vi "define.vi"(8 "error in (no error)":errorcluster, 11 "TrajectoryAK101022Resonance in":refnum<class "TrajectoryAK101022Resonance.lvclass">) -> (0 "error out":errorcluster, 3 "TrajectoryAK101022Resonance out":refnum<class "TrajectoryAK101022Resonance.lvclass">)   [LabVIEW 2010, in "TrajectoryAK101022Resonance.lvclass"]
doc: "modal dialog on which the user can set the trajectory parameters"
uses:
  TrajectoryAK101022Resonance.lvclass
  filter_type_enum.ctl
  TrajectoryAK101022Resonance.lvclass/TrajectoryAK101022Resonance.ctl
panel:
  out "frame rate":dbl[unit]
  out "resonance frequency":dbl[unit]
  out "Number of z points":i32
  out "repetitions (volumes)":i32
  out "number of planes":i32
  out "step size":dbl[unit]
  out "z signal":dbl[unit][][](graph)
  in  "Filter on?":bool
  in  "z-Function type":enum32{"Sine", "Stack", "Step"}(tab)
  out "ETL frequency":dbl[unit]=1.0 min=1.0
  in  "ETL amplitude conversion":dbl[unit]=500.0
  in  "ETL phase delay":dbl[unit]=0.008726646259971648
  in  "bi-directional?":bool
  in  "angle fraction":dbl=0.5
  out "Lines per z step (sine)":i32=1 caption="lines per z step" min=1
  in  "Level High (Step)":dbl caption="Level High"
  in  "Lines per z step (Step)":i32 caption="Lines per z step" min=1
  in  "Level overshoot (Step)":dbl caption="Level overshoot"
  in  "Level undershoot (Step)":dbl caption="Level undershoot"
  in  "Sample level high (Step)":u16 caption="Sample level high"
  in  "Sample overshoot (Step)":u16 caption="Sample overshoot"
  in  "Sample ramp (Step)":u16 caption="Sample ramp"
  in  "Sample undershoot (Step)":u16 caption="Sample undershoot"
  in  "filter type":T1
  in  "filter order":u16=2
  in  "low cutoff freq":dbl=0.125
  in  "high cutoff freq":dbl=0.45
  in  "button:cancel":bool
  in  "button:ok":bool
  # "Define TrajectoryAK101022Resonance"
  # "Filtering"
  # "In this mode, the z signal is sine function."
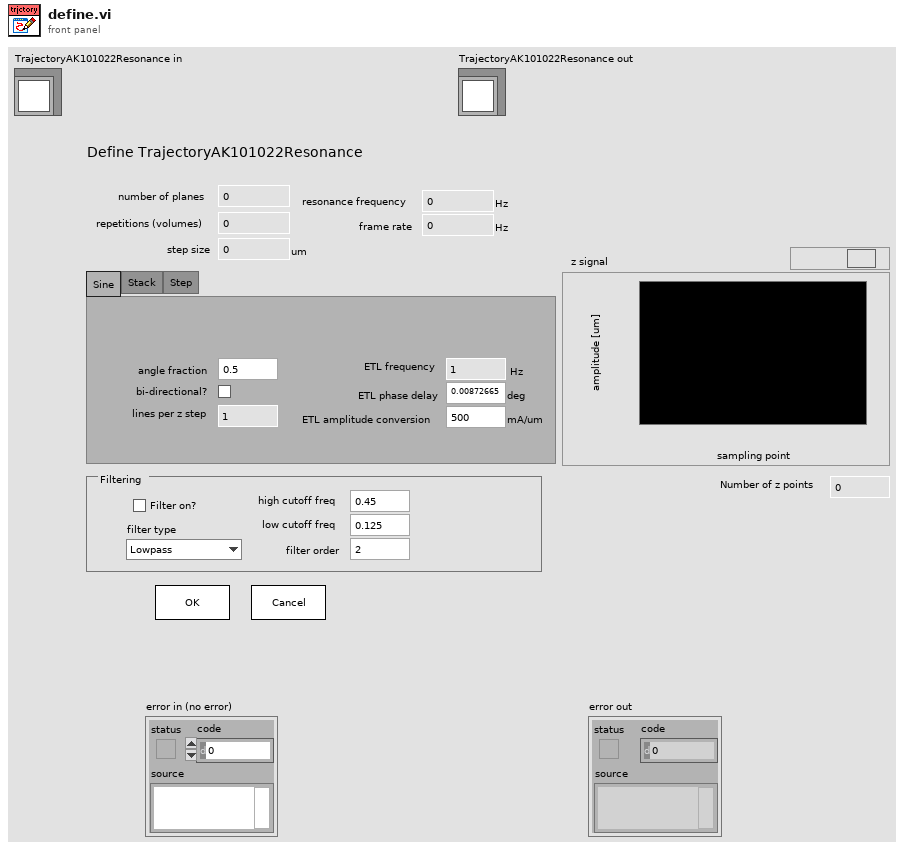
[diagram p1: front panel]
types:
  T1 = typedef "TrajectoryAK101022Resonance.lvclass/filter_type_enum.ctl" = enum16{"Lowpass", "Highpass", "Bandpass", "Bandstop"}
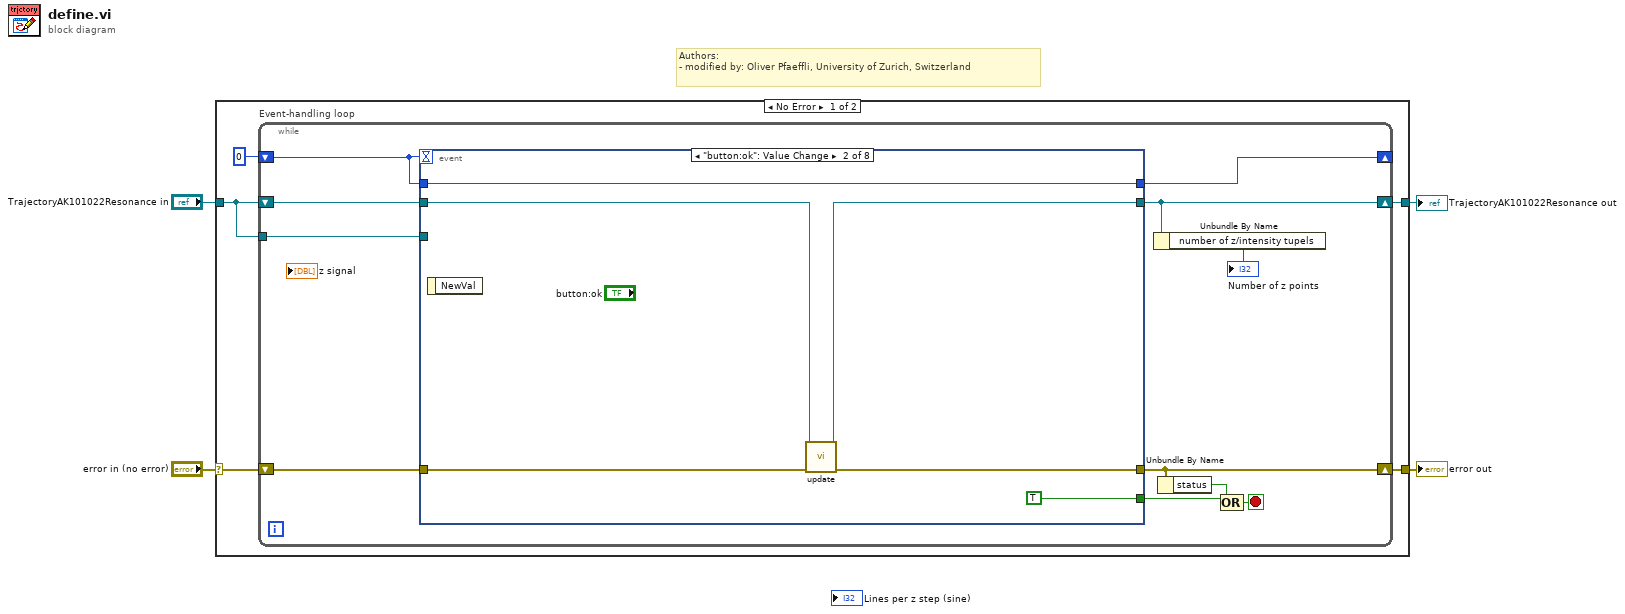
[diagram p0: block diagram]
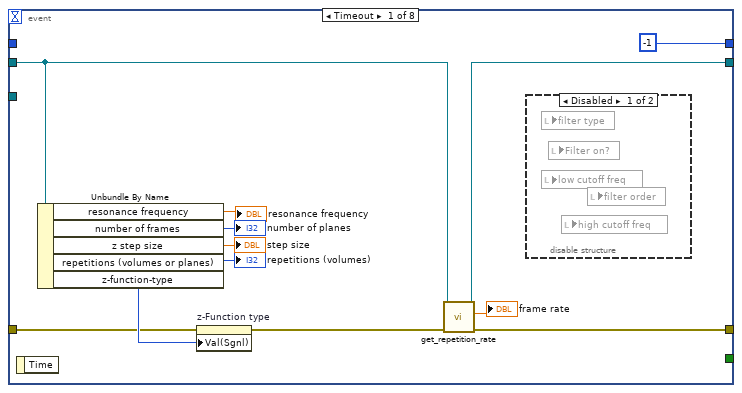
[diagram p2: hidden frame]
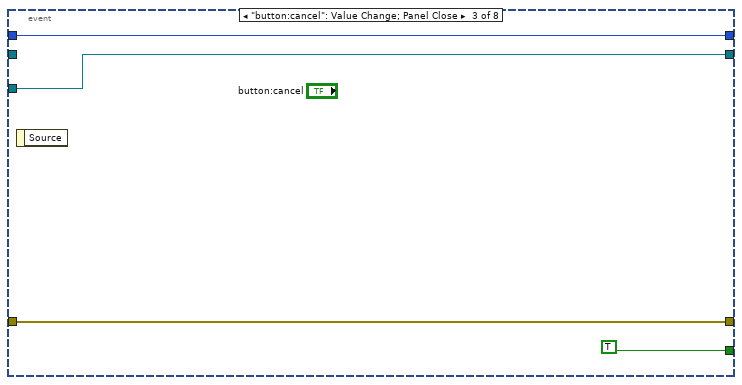
[diagram p4: hidden frame]
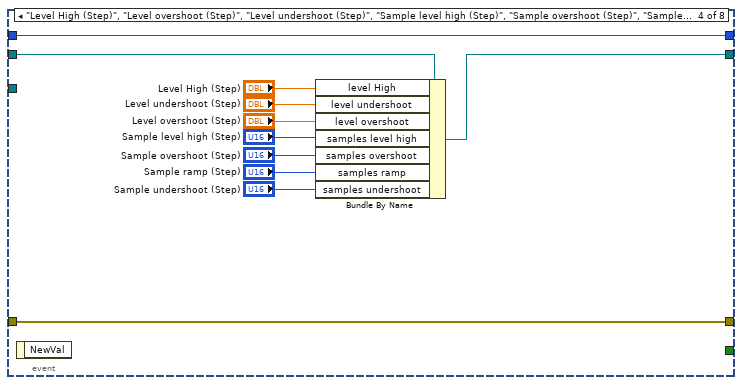
[diagram p5: hidden frame]
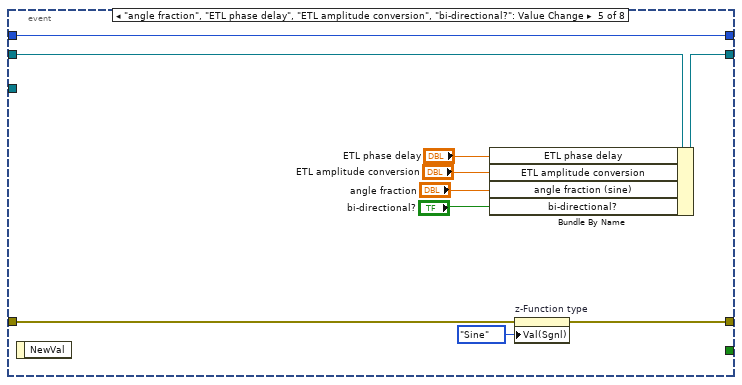
[diagram p6: hidden frame]
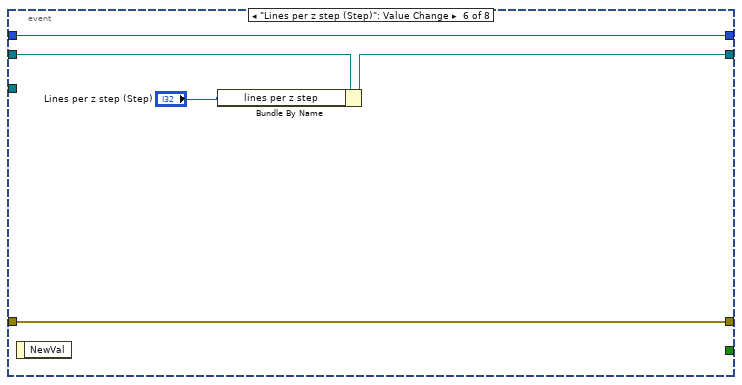
[diagram p7: hidden frame]
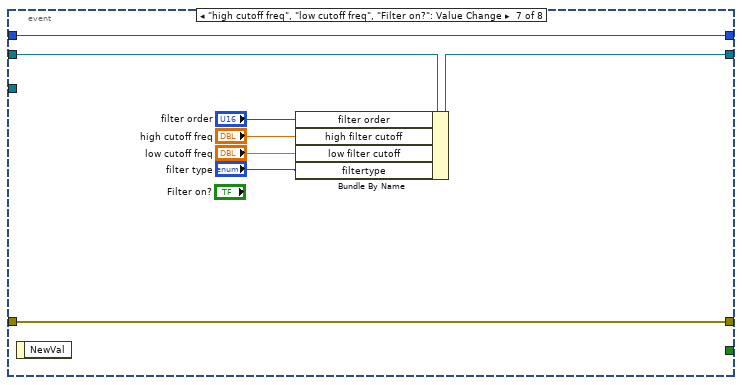
[diagram p8: hidden frame]
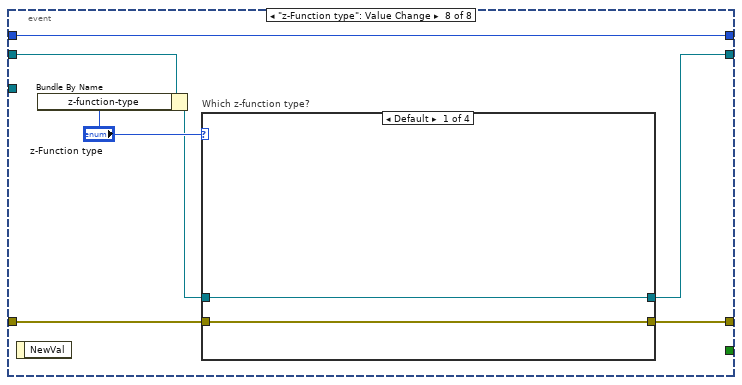
[diagram p9: hidden frame]
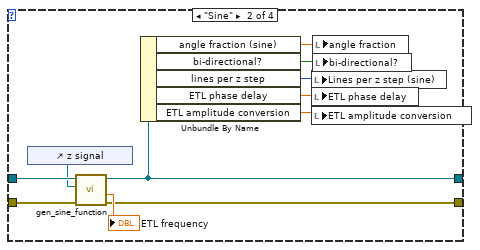
[diagram p10: hidden frame]
diagram:
  # "Authors: \n- modified by: Oliver Pfaeffli, University of Zurich, Switzerland"
  n1 = case shown="No Error" "error in (no error)" {
    selector: "error in (no error)" -> [w9 w102]
    tunnel: [w8 w102] -> w3
    tunnel: "TrajectoryAK101022Resonance in" -> [w5 w101]
    tunnel: [w7 w101] -> w1
    frame No Error {
      n2 = while "Event-handling loop" {
        shift-right: [w13] -> w8
        shift-left: w9 -> [w14]
        shift-right: [w16] -> _
        shift-left: 0 -> [w17]
        shift-right: [w11] -> w7
        shift-left: w5 -> [w18]
        tunnel: w5 -> [w15]
        stop <- w19 stop-if-true
        n3 = event shown="[1] \"button:ok\": Value Change" {
          selector: _ -> [_ _ _ _ _ _ _ _]
          dyn-events: _ -> [_ _ _ _ _ _ _ _]
          timeout: w17 -> [_ _ _ _ _ _ _ _]
          tunnel: w18 -> [w24 w33 _ w52 w54 w67 w75 w83]
          tunnel: w17 -> [_ w38 w42 w43 w63 w64 w69 w77]
          tunnel: [-1 w38 w42 w43 w63 w64 w69 w77] -> w16
          tunnel: [w27 w36 w41 w51 w62 w66 w74 w78] -> w11
          tunnel: w15 -> [_ _ w41 _ _ _ _ _]
          tunnel: w14 -> [w22 w34 w40 w53 w55 w68 w76 w82]
          tunnel: [w26 w35 w40 w53 w57 w68 w76 w81] -> w13
          tunnel: [_ TRUE TRUE _ _ _ _ _] -> w12
          event Timeout {
            n4 = event-data() -> ()  [unwired: 1 in, 1 out]
            n5 = Unbundle By Name(w24) -> ("resonance frequency"=→"resonance frequency":dbl[unit], "number of frames"=→"number of planes":i32, "z step size"=→"step size":dbl[unit], "repetitions (volumes or planes)"=→"repetitions (volumes)":i32, "z-function-type"=w23:enum16{"Sine", "Stack", "Step"})
            n6 = property on="z-Function type" class="TabCtl (strict)"(error in=w22, "Val(Sgnl)"=w23) -> (error out=w21:errorcluster)  [unwired: 1 in, 1 out]
            n7 = call-dynamic "get_repetition_rate.vi"("error in (no error)"=w21, "GenericTrajectory in"=w24) -> ("error out"=w26:errorcluster, "repetition rate"=→"frame rate":dbl[unit], "GenericTrajectory out"=w27:refnum<class "TrajectoryAK101022Resonance.lvclass">)  [unwired: 7 in]
            n8 = disable-structure shown="Disabled" {
              frame Disabled {
                n9 = local read "filter type"() -> ()  [unwired: 1 in]
                n10 = local read "low cutoff freq"() -> ()  [unwired: 1 in]
                n11 = local read "Filter on?"() -> ()  [unwired: 1 in]
                n12 = local read "high cutoff freq"() -> ()  [unwired: 1 in]
                n13 = local read "filter order"() -> ()  [unwired: 1 in]
              }
              frame Enabled {
              }
            }
          }
          event "button:ok": Value Change {
            n14 = event-data() -> ()  [unwired: 1 in, 1 out]
            n15 = call-dynamic "update.vi"("error in (no error)"=w34, "TrajectoryAK101022Resonance in"=w33) -> ("error out"=w35:errorcluster, "TrajectoryAK101022Resonance out"=w36:refnum<class "TrajectoryAK101022Resonance.lvclass">)  [unwired: 8 in]
          }
          event "button:cancel": Value Change; Panel Close {
            n16 = event-data() -> ()  [unwired: 1 in, 1 out]
          }
          event "Level High (Step)", "Level overshoot (Step)", "Level undershoot (Step)", "Sample level high (Step)", "Sample overshoot (Step)", "Sample ramp (Step)", "Sample undershoot (Step)": Value Change {
            n17 = event-data() -> ()  [unwired: 1 in, 1 out]
            n18 = Bundle By Name(cluster=w52, "level High"="Level High (Step)", "level undershoot"="Level undershoot (Step)", "level overshoot"="Level overshoot (Step)", "samples level high"="Sample level high (Step)", "samples overshoot"="Sample overshoot (Step)", "samples ramp"="Sample ramp (Step)", "samples undershoot"="Sample undershoot (Step)") -> (w51:refnum<class "TrajectoryAK101022Resonance.lvclass">)
          }
          event "angle fraction", "ETL phase delay", "ETL amplitude conversion", "bi-directional?": Value Change {
            n19 = event-data() -> ()  [unwired: 1 in, 1 out]
            n20 = Bundle By Name(cluster=w54, "ETL phase delay"="ETL phase delay", "ETL amplitude conversion"="ETL amplitude conversion", "angle fraction (sine)"="angle fraction", "bi-directional?"="bi-directional?") -> (w62:refnum<class "TrajectoryAK101022Resonance.lvclass">)
            n21 = property on="z-Function type" class="TabCtl (strict)"(error in=w55, "Val(Sgnl)"=enum32{"Sine", "Stack", "Step"}."Sine" ("Value (Signaling)")) -> (error out=w57:errorcluster)  [unwired: 1 in, 1 out]
          }
          event "Lines per z step (Step)": Value Change {
            n22 = event-data() -> ()  [unwired: 1 in, 1 out]
            n23 = Bundle By Name(cluster=w67, "lines per z step"="Lines per z step (Step)") -> (w66:refnum<class "TrajectoryAK101022Resonance.lvclass">)
          }
          event "high cutoff freq", "low cutoff freq", "Filter on?": Value Change {
            n24 = event-data() -> ()  [unwired: 1 in, 1 out]
            n25 = Bundle By Name(cluster=w75, "filter order"="filter order", "high filter cutoff"="high cutoff freq", "low filter cutoff"="low cutoff freq", "filtertype"="filter type") -> (w74:refnum<class "TrajectoryAK101022Resonance.lvclass">)
          }
          event "z-Function type": Value Change {
            n26 = event-data() -> ()  [unwired: 1 in, 1 out]
            n27 = Bundle By Name(cluster=w83, "z-function-type"="z-Function type") -> (w79:refnum<class "TrajectoryAK101022Resonance.lvclass">)
            n28 = case "Which z-function type?" shown="Default" "z-Function type" {
              tunnel: w82 -> [w85 w95 w98 w100]
              tunnel: [w85 w94 w98 w100] -> w81
              tunnel: w79 -> [w84 w93 w97 w99]
              tunnel: [w84 w90 w97 w99] -> w78
              frame Default {
              }
              frame "Sine" {
                n29 = control-ref of="z signal"() -> (w86:refnum<vi>)
                n30 = call "gen_sine_function.vi"("error in (no error)"=w95, "z signal graph ref"=w86, "TrajectoryAK101022Resonance in"=w93) -> ("error out"=w94:errorcluster, "z-frequency"=→"ETL frequency":dbl[unit], "TrajectoryAK101022Resonance out"=w90:refnum<class "TrajectoryAK101022Resonance.lvclass">)  [unwired: 5 in, 1 out]
                n31 = Unbundle By Name(w90) -> ("angle fraction (sine)"=w92:dbl, "bi-directional?"=w91:bool, "lines per z step"=w89:i32, "ETL phase delay"=w88:dbl[unit], "ETL amplitude conversion"=w87:dbl[unit])
                n32 = local write "Lines per z step (sine)"(w89) -> ()
                n33 = local write "ETL phase delay"(w88) -> ()
                n34 = local write "ETL amplitude conversion"(w87) -> ()
                n35 = local write "angle fraction"(w92) -> ()
                n36 = local write "bi-directional?"(w91) -> ()
              }
              frame "Stack" {
              }
              frame "Step" {
              }
            }
          }
        }
        n37 = Unbundle By Name(w11) -> ("number of z/intensity tupels"=→"Number of z points":i32)
        n38 = Unbundle By Name(w13) -> ("status"=w20:bool)
        n39 = Compound Arithmetic op=OR(w20, w12) -> (w19:bool)
      }
    }
    frame Error {
    }
  }
  "error out" <- w3
  "TrajectoryAK101022Resonance out" <- w1
